vi "G-Code Parser.vi"(8 "Error In":errorcluster, 11 "G Code File Path":path) -> (0 "Error Out":errorcluster, 1 "Ready":bool, 2 "G Code Commands":T1[](array[typedef]))   [LabVIEW 2018]
doc: "This GCode parser extracts the GCode commands into an \"Command Array\". Command Array contains the parameters for each command."
uses:
  Type Defs/G Code Command Cluster.ctl
panel:
  out "Number of lines read":i32
  # "USE EOL as end."
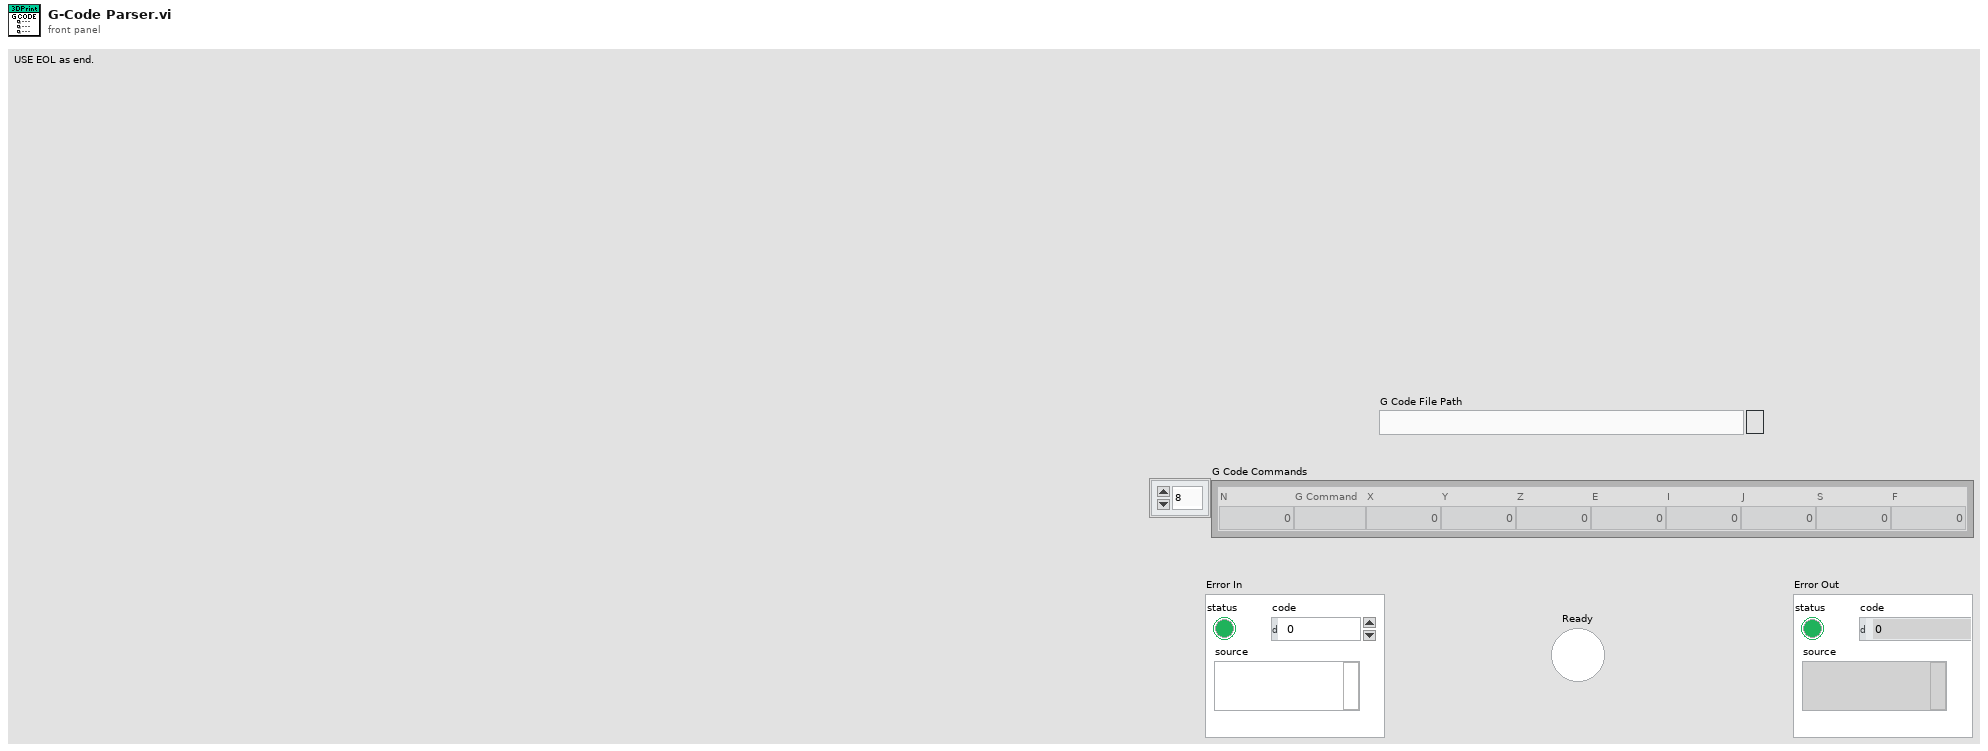
[diagram p1: front panel]
types:
  T1 = typedef "G Code Command Cluster.ctl" = cluster{"N":dbl, "G Command":string, "X":dbl, "Y":dbl, "Z":dbl, "E":dbl, "I":dbl, "J":dbl, "S":dbl, "F":dbl}
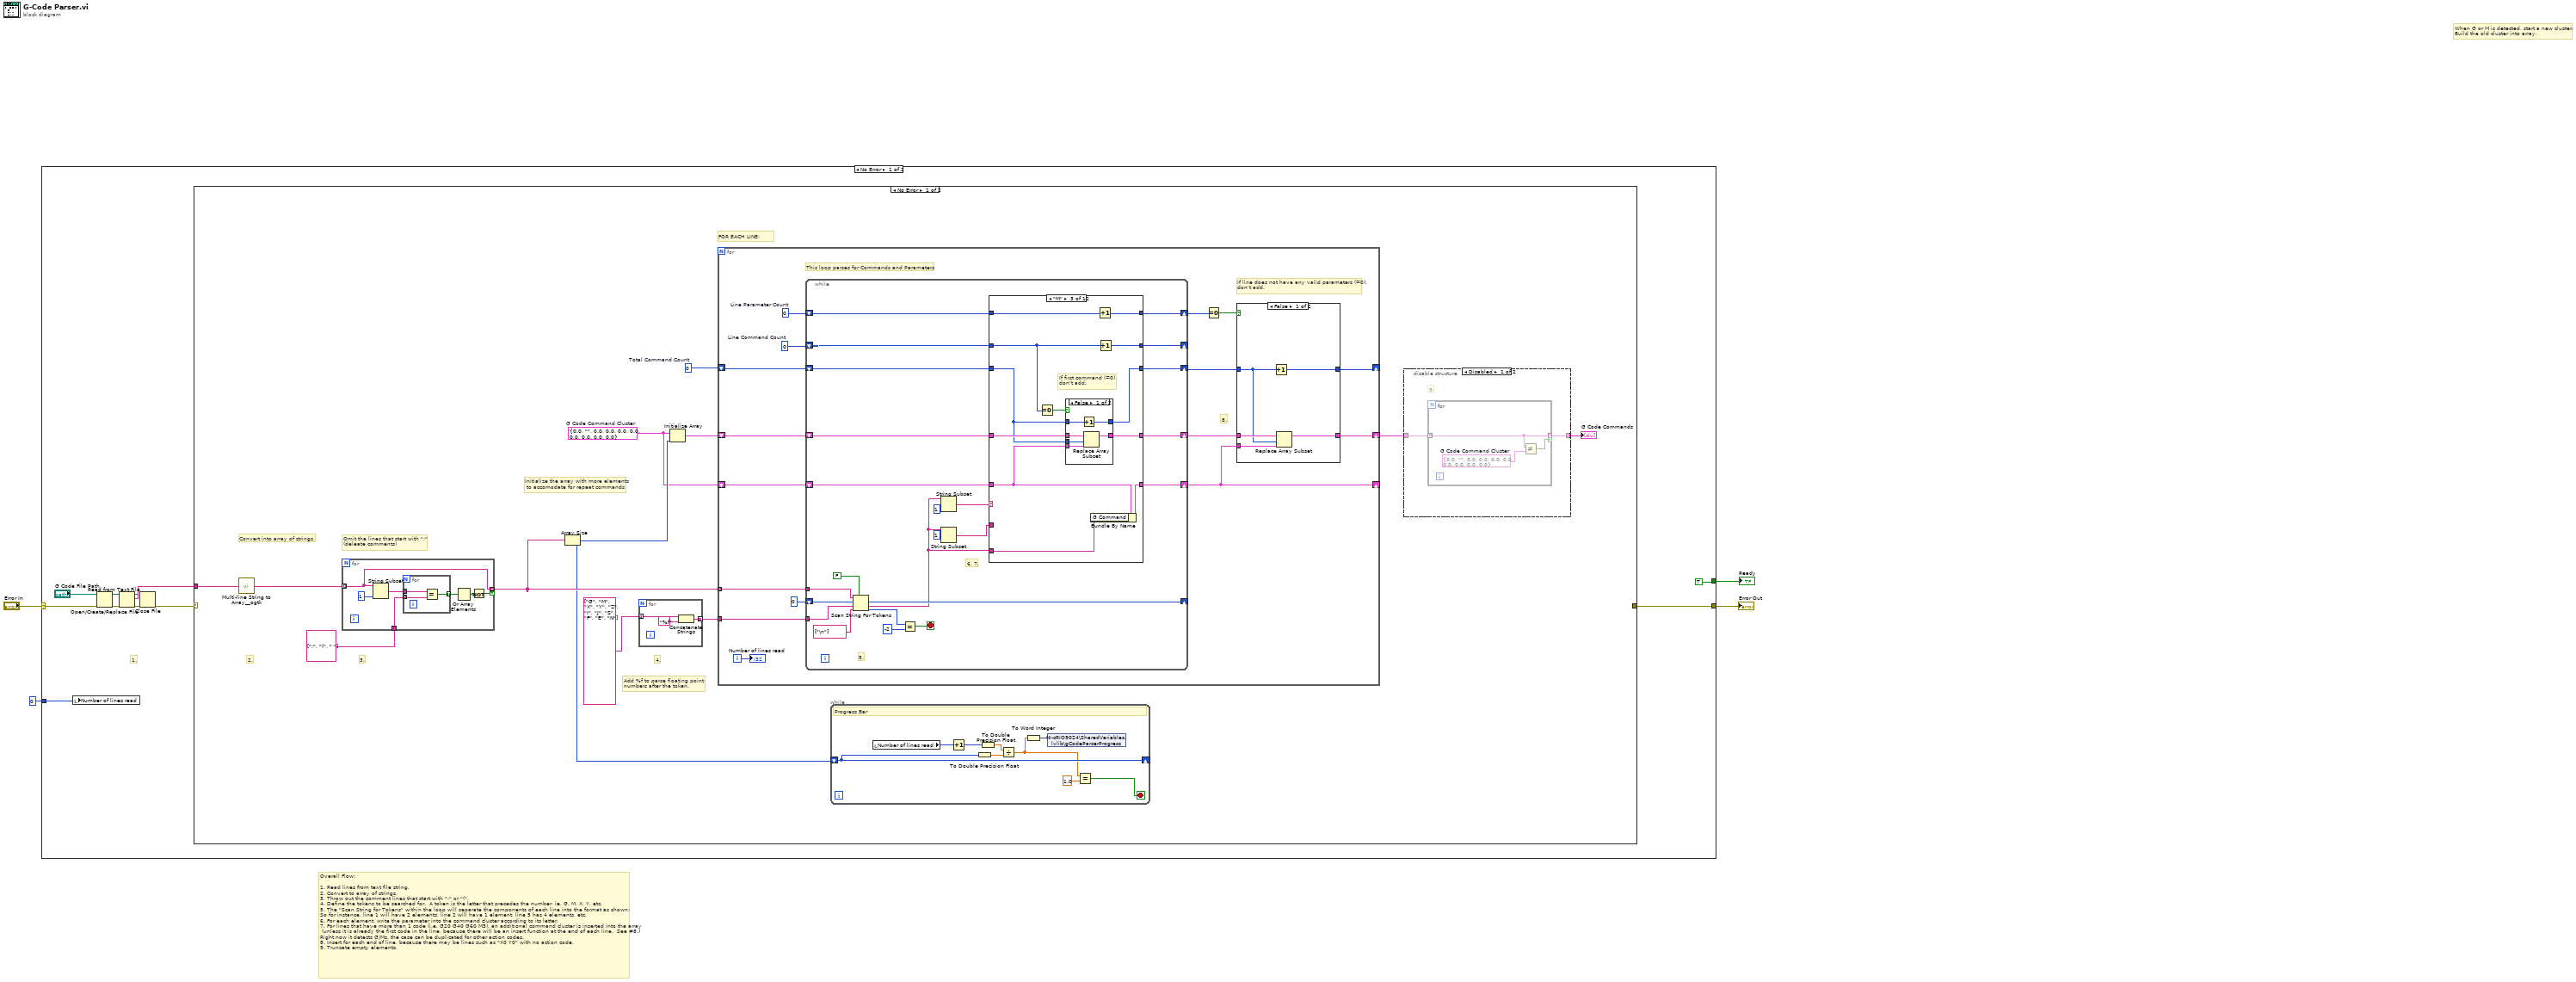
[diagram p0: block diagram]
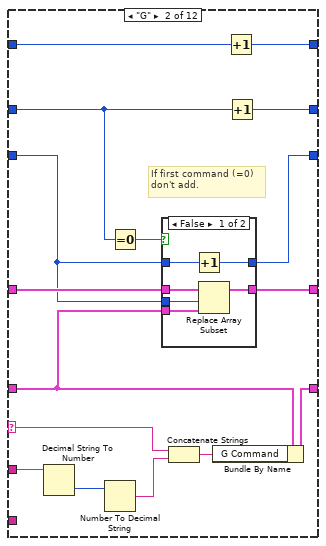
[diagram p5: hidden frame]
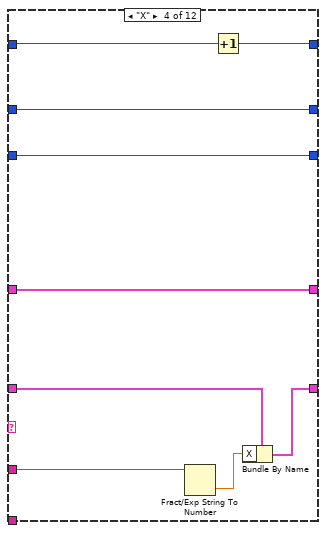
[diagram p8: hidden frame]
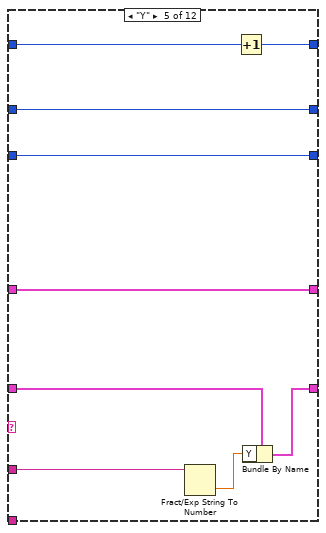
[diagram p9: hidden frame]
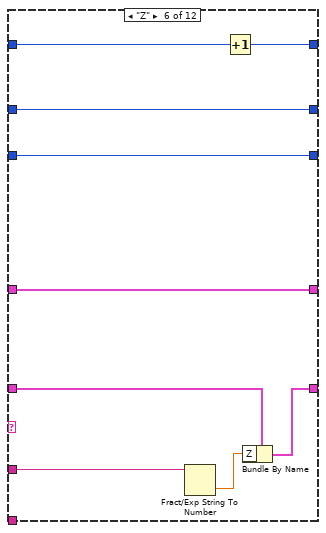
[diagram p10: hidden frame]
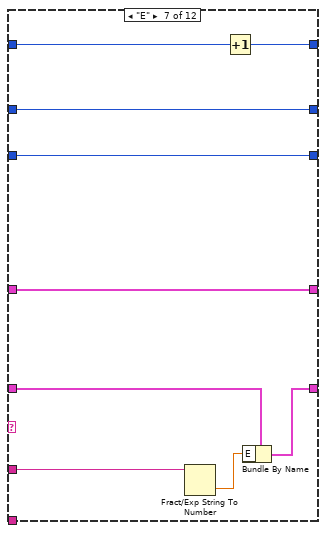
[diagram p11: hidden frame]
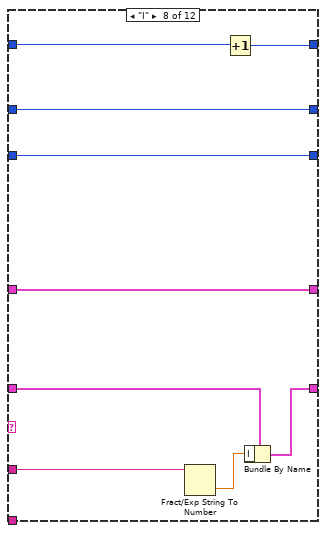
[diagram p12: hidden frame]
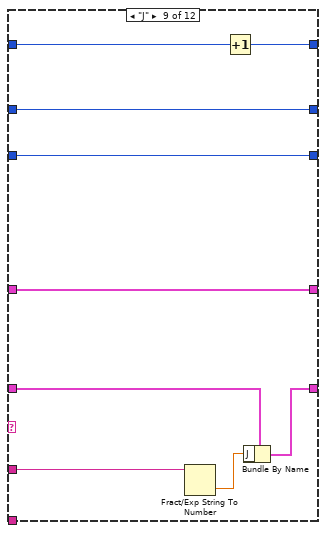
[diagram p13: hidden frame]
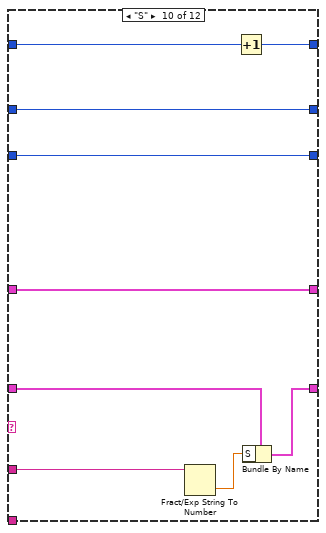
[diagram p14: hidden frame]
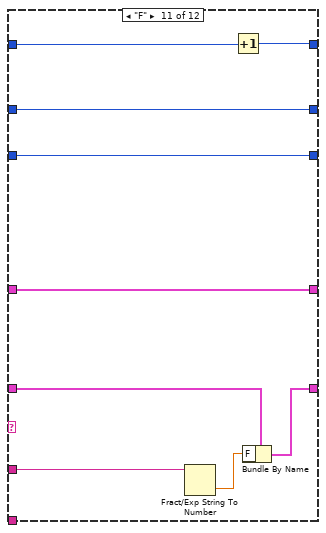
[diagram p15: hidden frame]
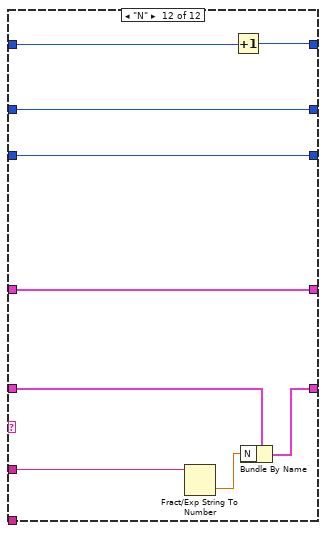
[diagram p16: hidden frame]
diagram:
  # "Overall Flow:\n\n1.\tRead lines from text file string.\n2.\tConvert to array of strings.\n3.\tThrow out the comment lines that start with \";\" or \"(\". \n4.\tDefine the tokens to be searched for.  A token is the letter that precedes the number, ie. G, M, X, Y, etc.\n5.\tThe \"Scan String for Tokens\" within the loop will separate the components of each line into the format as shown: \nSo for instance, line 1 will have 2 elements, line 2 will have 1 element, line 5 has 4 elements, etc.\n6.\tFor each element, write the parameter into the command cluster according to its letter.\n7.\tFor lines that have more than 1 code (i.e. G20 G40 G60 M3), an additional command cluster is inserted into the array\n (unless it is already the first code in the line, because there will be an insert function at the end of each line.  See #8.)  \nRight now it detects G/Ms, the case can be duplicated for other action codes.\n8.\tInsert for each end of line, because there may be lines such as \"X0 Y0\" with no action code.\n9. Truncate empty elements."
  # "When G or M is detected, start a new cluster.\nBuild the old cluster into array."
  n1 = case shown="No Error" "Error In" {
    selector: "Error In" -> [w14 w234]
    tunnel: [w7 w234] -> w3
    tunnel: 0 ("Number of lines read") -> [w6 _]
    tunnel: [TRUE _] -> w1
    frame No Error {
      # "1."
      n2 = local write "Number of lines read"(w6) -> ()
      n3 = Open/Create/Replace File(file path (use dialog)="G Code File Path", error in=w14) -> (refnum out=w12:refnum<file>, error out=w13:errorcluster)  [unwired: 4 in, 1 out]
      n4 = Read from Text File(file (use dialog)=w12, error in=w13) -> (refnum out=w10:refnum<file>, text=w15:string, error out=w11:errorcluster)  [unwired: 2 in, 1 out]
      n5 = Close File(refnum=w10, error in=w11) -> (error out=w8:errorcluster)  [unwired: 1 out]
      n6 = case shown="No Error" w8 {
        selector: w8 -> [_ w233]
        tunnel: w15 -> [w19 _]
        tunnel: [_ w233] -> w7
        frame No Error {
          w17 = T1 {"N"=0.0, "G Command"="", "X"=0.0, "Y"=0.0, "Z"=0.0, "E"=0.0, "I"=0.0, "J"=0.0, "S"=0.0, "F"=0.0}  # G Code Command Cluster
          w23 = 0  # Total Command Count
          # "Initialize the array with more elements\n to accomodate for repeat commands"
          # "Convert into array of strings."
          # "4."
          # "3."
          # "2."
          # "Add %f to parse floating point \nnumbers after the token."
          # "FOR EACH LINE:"
          # "Omit the lines that start with \";\"\n(deleate comments)"
          n7 = call <userlib>:"Multi-line String to Array__ogtk.vi"("string"=w19) -> ("lines"=w27:string[])
          n8 = for {
            tunnel: w27 -> [w227] mode=indexing
            tunnel: [w227] -> w22 mode=indexing if=w228
            tunnel: string[] [";", "(", " "] ("Comment char") -> [w226]
            n9 = String Subset(string=w227, length (rest)=1 ("length (rest)")) -> (substring=w225:string)  [unwired: 1 in]
            n10 = for {
              tunnel: w226 -> [w231] mode=indexing
              tunnel: w225 -> [w232]
              tunnel: [w230] -> w224 mode=indexing
              n11 = Equal?(x=w232, y=w231) -> (x = y?=w230:bool)
            }
            n12 = Or Array Elements(Boolean array=w224) -> (logical OR=w223:bool)
            n13 = Not(x=w223) -> (.not. x?=w228:bool)
          }
          n14 = Array Size(array=w22) -> (size(s)=w18:i32)
          n15 = for {
            tunnel: string[] ["G", "M", "X", "Y", "Z", "I", "J", "S", "F", "E", "N"] ("Search Tokens") -> [w45] mode=indexing
            tunnel: [w43] -> w25 mode=indexing
            n16 = Concatenate Strings(w45, "%f" ("string")) -> (w43:string)
          }
          n17 = Initialize Array "Initialize Array"(w17, w18) -> (w24:T1[])
          n18 = for {
            tunnel: w22 -> [w60] mode=indexing
            shift-right: [w51] -> _
            shift-left: w17 -> [w59]
            tunnel: w25 -> [w58]
            shift-right: [w47] -> w21
            shift-left: w24 -> [w57]
            shift-right: [w52] -> _
            shift-left: w23 -> [w55]
            i -> [w46]
            w49 = 0  # Line Parameter Count
            w56 = 0  # Line Command Count
            # "8."
            # "If line does not have any valid parameters (=0),\ndon't add."
            # "This loop parses for Commands and Parameters"
            n19 = while {
              tunnel: w58 -> [w92]
              tunnel: w60 -> [w87]
              shift-right: [w90] -> _
              shift-left: 0 ("offset past token") -> [w91]
              shift-right: [w82] -> w51
              shift-left: w59 -> [w76]
              shift-right: [w77] -> w54
              shift-left: w57 -> [w73]
              shift-right: [w78] -> _
              shift-left: w56 -> [w79]
              shift-right: [w75] -> w53
              shift-left: w55 -> [w74]
              shift-right: [w70] -> w48
              shift-left: w49 -> [w71]
              stop <- w81 stop-if-true
              # "6, 7."
              # "5."
              n20 = Scan String For Tokens(5:FALSE ("allow empty tokens? (F)"), 6:string[] ["\n"] ("delimiters (\\s,\\t,\\r,\\n)"), 7:w92, 8:w91, 9:w87) -> (0:w88:i32, 1:w69:string, 2:w90:i32)  [unwired: 1 in, 1 out]
              n21 = Equal?(x=w88, y=-2) -> (x = y?=w81:bool)
              n22 = String Subset(string=w69, length (rest)=1 ("length (rest)")) -> (substring=w84:string)  [unwired: 1 in]
              n23 = String Subset(string=w69, offset (0)=1) -> (substring=w83:string)  [unwired: 1 in]
              n24 = case shown="\"M\"" w84 {
                selector: w84 -> [_ w99 _ _ _ _ _ _ _ _ _ _]
                tunnel: [w97 w113 w133 w150 w159 w168 w177 w186 w195 w204 w213 w222] -> w82
                tunnel: w83 -> [_ w102 _ w148 w157 w166 w175 w184 w193 w202 w211 w220]
                tunnel: w76 -> [w97 w109 w128 w147 w156 w165 w174 w183 w192 w201 w210 w219]
                tunnel: w69 -> [_ _ w132 _ _ _ _ _ _ _ _ _]
                tunnel: w79 -> [w96 w110 w129 w146 w155 w164 w173 w182 w191 w200 w209 w218]
                tunnel: [w96 w108 w127 w146 w155 w164 w173 w182 w191 w200 w209 w218] -> w78
                tunnel: w73 -> [w95 w111 w130 w145 w154 w163 w172 w181 w190 w199 w208 w217]
                tunnel: [w95 w112 w131 w145 w154 w163 w172 w181 w190 w199 w208 w217] -> w77
                tunnel: w74 -> [w94 w107 w126 w144 w153 w162 w171 w180 w189 w198 w207 w216]
                tunnel: [w94 w106 w125 w144 w153 w162 w171 w180 w189 w198 w207 w216] -> w75
                tunnel: w71 -> [w93 w104 w123 w143 w152 w161 w170 w179 w188 w197 w206 w215]
                tunnel: [w93 w103 w122 w142 w151 w160 w169 w178 w187 w196 w205 w214] -> w70
                frame Default {
                }
                frame "G" {
                  # "If first command (=0)\ndon't add."
                  n25 = Decimal String To Number(string=w102) -> (number=w101:i32)  [unwired: 2 in, 1 out]
                  n26 = Number To Decimal String(number=w101) -> (decimal integer string=w100:string)  [unwired: 1 in]
                  n27 = Equal To 0?(x=w110) -> (x = 0?=w105:bool)
                  n28 = case shown="False" w105 {
                    tunnel: w109 -> [w119 _]
                    tunnel: [w117 w121] -> w112
                    tunnel: w111 -> [w118 w121]
                    tunnel: w107 -> [w116 _]
                    tunnel: w107 -> [w115 w120]
                    tunnel: [w114 w120] -> w106
                    frame False {
                      n29 = Increment(x=w115) -> (x+1=w114:i32)
                      n30 = Replace Array Subset(array=w118, new element=w119, index=w116) -> (w117:T1[])
                    }
                    frame True {
                    }
                  }
                  n31 = Concatenate Strings(w99, w100) -> (w98:string)
                  n32 = Bundle By Name(cluster=w109, "G Command"=w98) -> (w113:T1)
                  n33 = Increment(x=w104) -> (x+1=w103:i32)
                  n34 = Increment(x=w110) -> (x+1=w108:i32)
                }
                frame "M" {
                  # "If first command (=0)\ndon't add."
                  n35 = Equal To 0?(x=w129) -> (x = 0?=w124:bool)
                  n36 = case shown="False" w124 {
                    tunnel: w128 -> [w139 _]
                    tunnel: [w137 w141] -> w131
                    tunnel: w130 -> [w138 w141]
                    tunnel: w126 -> [w136 _]
                    tunnel: w126 -> [w135 w140]
                    tunnel: [w134 w140] -> w125
                    frame False {
                      n37 = Increment(x=w135) -> (x+1=w134:i32)
                      n38 = Replace Array Subset(array=w138, new element=w139, index=w136) -> (w137:T1[])
                    }
                    frame True {
                    }
                  }
                  n39 = Bundle By Name(cluster=w128, "G Command"=w132) -> (w133:T1)
                  n40 = Increment(x=w123) -> (x+1=w122:i32)
                  n41 = Increment(x=w129) -> (x+1=w127:i32)
                }
                frame "X" {
                  n42 = Fract/Exp String To Number(string=w148) -> (number=w149:dbl)  [unwired: 3 in, 1 out]
                  n43 = Increment(x=w143) -> (x+1=w142:i32)
                  n44 = Bundle By Name(cluster=w147, "X"=w149) -> (w150:T1)
                }
                frame "Y" {
                  n45 = Fract/Exp String To Number(string=w157) -> (number=w158:dbl)  [unwired: 3 in, 1 out]
                  n46 = Increment(x=w152) -> (x+1=w151:i32)
                  n47 = Bundle By Name(cluster=w156, "Y"=w158) -> (w159:T1)
                }
                frame "Z" {
                  n48 = Fract/Exp String To Number(string=w166) -> (number=w167:dbl)  [unwired: 3 in, 1 out]
                  n49 = Increment(x=w161) -> (x+1=w160:i32)
                  n50 = Bundle By Name(cluster=w165, "Z"=w167) -> (w168:T1)
                }
                frame "E" {
                  n51 = Fract/Exp String To Number(string=w175) -> (number=w176:dbl)  [unwired: 3 in, 1 out]
                  n52 = Increment(x=w170) -> (x+1=w169:i32)
                  n53 = Bundle By Name(cluster=w174, "E"=w176) -> (w177:T1)
                }
                frame "I" {
                  n54 = Fract/Exp String To Number(string=w184) -> (number=w185:dbl)  [unwired: 3 in, 1 out]
                  n55 = Increment(x=w179) -> (x+1=w178:i32)
                  n56 = Bundle By Name(cluster=w183, "I"=w185) -> (w186:T1)
                }
                frame "J" {
                  n57 = Fract/Exp String To Number(string=w193) -> (number=w194:dbl)  [unwired: 3 in, 1 out]
                  n58 = Increment(x=w188) -> (x+1=w187:i32)
                  n59 = Bundle By Name(cluster=w192, "J"=w194) -> (w195:T1)
                }
                frame "S" {
                  n60 = Fract/Exp String To Number(string=w202) -> (number=w203:dbl)  [unwired: 3 in, 1 out]
                  n61 = Increment(x=w197) -> (x+1=w196:i32)
                  n62 = Bundle By Name(cluster=w201, "S"=w203) -> (w204:T1)
                }
                frame "F" {
                  n63 = Fract/Exp String To Number(string=w211) -> (number=w212:dbl)  [unwired: 3 in, 1 out]
                  n64 = Increment(x=w206) -> (x+1=w205:i32)
                  n65 = Bundle By Name(cluster=w210, "F"=w212) -> (w213:T1)
                }
                frame "N" {
                  n66 = Fract/Exp String To Number(string=w220) -> (number=w221:dbl)  [unwired: 3 in, 1 out]
                  n67 = Increment(x=w215) -> (x+1=w214:i32)
                  n68 = Bundle By Name(cluster=w219, "N"=w221) -> (w222:T1)
                }
              }
            }
            n69 = Equal To 0?(x=w48) -> (x = 0?=w50:bool)
            n70 = case shown="False" w50 {
              tunnel: w54 -> [w66 w67]
              tunnel: w51 -> [w65 _]
              tunnel: [w64 w68] -> w52
              tunnel: w53 -> [w63 w68]
              tunnel: [w62 w67] -> w47
              frame False {
                n71 = Increment(x=w63) -> (x+1=w64:i32)
                n72 = Replace Array Subset "Replace Array Subset"(array=w66, new element=w65, index=w63) -> (w62:T1[])
              }
              frame True {
              }
            }
            "Number of lines read" <- w46
          }
          n73 = while {
            shift-right: [w36] -> _
            shift-left: w18 -> [w36]
            stop <- w37 stop-if-true
            # "Progress Bar"
            n74 = local read "Number of lines read"() -> (w42:i32)
            n75 = Increment(x=w42) -> (x+1=w39:i32)
            n76 = To Double Precision Float(number=w36) -> (double precision float=w41:dbl)
            n77 = To Double Precision Float(number=w39) -> (double precision float=w40:dbl)
            n78 = Divide(x=w40, y=w41) -> (x/y=w34:dbl)
            n79 = To Word Integer(number=w34) -> (16bit integer=w35:i16)
            n80 = shared-variable "NI-cRIO9024\\SharedVariables.lvlib\\gCodeParserProgress"(w35) -> ()  [unwired: 1 in, 1 out]
            n81 = Equal?(x=w34, y=1.0) -> (x = y?=w37:bool)
          }
          n82 = disable-structure shown="Disabled" {
            disable-tunnel: w21 -> [w29 w33]
            disable-tunnel: [w28 w33] -> w16
            frame Disabled {
              # "9."
              n83 = for {
                tunnel: w29 -> [w32] mode=indexing
                tunnel: [w32] -> w28 mode=indexing if=w31
                w30 = T1 {"N"=0.0, "G Command"="", "X"=0.0, "Y"=0.0, "Z"=0.0, "E"=0.0, "I"=0.0, "J"=0.0, "S"=0.0, "F"=0.0}  # G Code Command Cluster
                n84 = Not Equal?(x=w32, y=w30) -> (x != y?=w31:bool)
              }
            }
            frame Enabled {
            }
          }
          "G Code Commands" <- w16
        }
        frame Error {
        }
      }
    }
    frame Error {
    }
  }
  "Error Out" <- w3
  "Ready" <- w1
